vi "Initialize New.vi"(4 "Error In":errorcluster, 7 "Config Data in":refnum<class "Config Data.lvclass">) -> (0 "Error Out":errorcluster, 3 "Config Data out":refnum<class "Config Data.lvclass">)   [LabVIEW 2014, in "Config Data.lvlib" / "Config Data.lvclass"]
uses:
  Config Data.lvclass
  Config Data.lvclass/Config Data.ctl
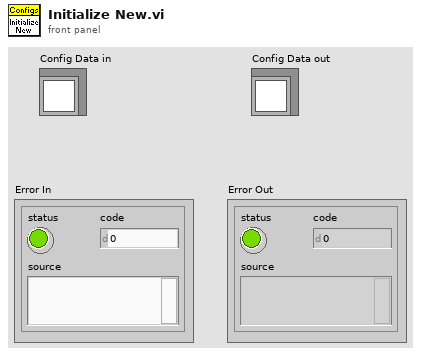
[diagram p1: front panel]
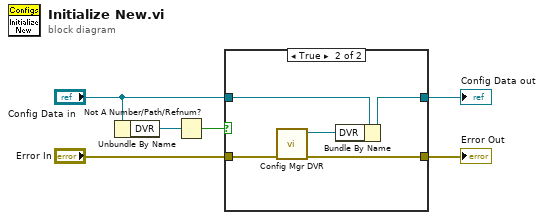
[diagram p0: block diagram]
diagram:
  n1 = Unbundle By Name("Config Data in") -> ("DVR"=w6:refnum<data-value>)
  n2 = Not A Number/Path/Refnum?(number/path/refnum=w6) -> (NaN/Path/Refnum?=w5:bool)
  n3 = case shown="True" w5 {
    tunnel: "Config Data in" -> [w8 w13]
    tunnel: [w8 w12] -> w3
    tunnel: "Error In" -> [w7 w11]
    tunnel: [w7 w9] -> w1
    frame False {
    }
    frame True {
      n4 = call "Config Mgr DVR.vi"("Error In"=w11) -> ("Error Out"=w9:errorcluster, "DVR"=w10:refnum<data-value>)  [unwired: 5 in]
      n5 = Bundle By Name(cluster=w13, "DVR"=w10) -> (w12:refnum<class "Config Data.lvclass">)
    }
  }
  "Error Out" <- w1
  "Config Data out" <- w3
